vi "Read Mask Paramter.vi"(7 "Type":T2, 11 "AllProcessSettingOut":T3[](array[typedef])) -> (3 "data":T1)   [LabVIEW 2019]
uses:
  Controls/MaskParam_Type.ctl
  Controls/Process_Type.ctl
  Controls/Process_Setting.ctl
  Ctrl/VisionProcessName.ctl
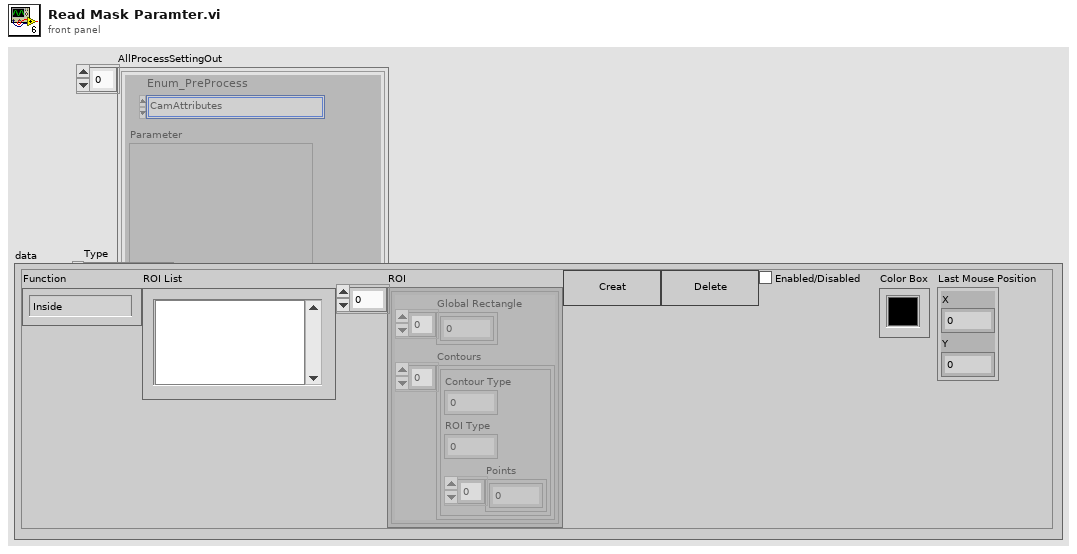
[diagram p1: front panel]
types:
  T1 = typedef "MaskParam_Type.ctl" = cluster{"Function":enum16{"Inside", "Outside"}, "ROI List":i32, "ROI":cluster{"Global Rectangle":i32[], "Contours":cluster{"Contour Type":u32, "ROI Type":u32, "Points":i32[]}[]}[], "Creat ROI":bool, "Delete ROI":bool, "Enabled/Disabled":bool, "Color Box":u32, "Last Mouse Position":cluster{"X":i32, "Y":i32}}
  T2 = typedef "Process_Type.ctl" = enum16{"None", "ExtractPlane", "BinaryMono", "Operators", "GrayMorphology", "Filters", "Lookup Table", "Particle Filter", "Mask"}
  T3 = typedef "Process_Setting.ctl" = cluster{"Enum_PreProcess":T4, "Parameter":string}
  T4 = typedef "VisionProcessName.ctl" = enum16{"*CamParameter*", "CamAttributes", "*Preprocess*", "CG_Brightness", "C_Plane Extraction", "C_Threshold", "G_Lookup Table", "G_Threshold"}
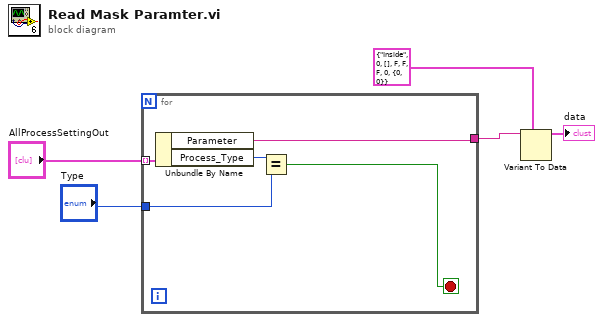
[diagram p0: block diagram]
diagram:
  n1 = for {
    tunnel: "AllProcessSettingOut" -> [w10] mode=indexing
    tunnel: "Type" -> [w8]
    tunnel: [w6] -> w3
    stop <- w7 stop-if-true
    n2 = Unbundle By Name(w10) -> ("Parameter"=w6:string, "Process_Type"=w9:T2)
    n3 = Equal?(x=w9, y=w8) -> (x = y?=w7:bool)
  }
  n4 = Variant To Data(type=T1 {"Function"=enum."Inside", "ROI List"=0, "ROI"=[], "Creat ROI"=FALSE, "Delete ROI"=FALSE, "Enabled/Disabled"=FALSE, "Color Box"=0, "Last Mouse Position"={"X"=0, "Y"=0}} ("MaskParam"), Variant=w3) -> (data=→"data":T1)  [unwired: 1 in, 1 out]
